vi "Transmit Messages with Rate-based Schedule.vi"() -> ()   [LabVIEW 2023]
doc: "This program opens the specified card, builds a transmit schedule \nusing transmit interval information in the channel configuration file,\nand then transmits the messages with changing data."
uses:
  <instrlib>/BTICardLib/Private/Initialize By Card Number and Core Number.vi
  <instrlib>/BTICardLib/Private/Configure Core From XML.vi
  <instrlib>/BTI429Lib/Private/Tx/Configure/Configure Tx Channel From XML.vi
  <instrlib>/BTI429Lib/Private/Core/Action-Status/Start Channel.vi
  <instrlib>/BTI429Lib/Private/Utility/Get BNR Sign.vi
  <instrlib>/BTI429Lib/Private/Utility/Get BNR Data.vi
  <instrlib>/BTI429Lib/Private/Utility/Get BNR Val.vi
  <instrlib>/BTI429Lib/Private/Utility/Get BNR Mantissa.vi
  <instrlib>/BTI429Lib/Private/Utility/Get BNR SSM.vi
  <instrlib>/BTI429Lib/Private/Utility/Set BNR Mantissa.vi
  <instrlib>/BTI429Lib/Private/Core/Action-Status/Stop Channel.vi
  <instrlib>/BTICardLib/BTICardLV.lvlib
  <instrlib>/BTI429Lib/BTI429LV.lvlib
panel:
  in  "Channel Configuration XML file name":string="Channel Config.xml"
  in  "Core Configuration XML file name":string="Core Config.xml"
  in  "Card Number":i32
  in  "Channel Number":i32=16
  in  "Core Number":i32
  out "Core Xml Path":path
  out "Channel Xml Path":path
  out "twosmantissaout":u32
  out "NEW sign out":u16
  in  "TwosComplement":u16
  out "message out":u32 format="%.0b"
  out "mantissa out":u32 format="%.0b"
  out "sign/status matrix (SSM)":u16 format="%1b"
  out "Data-NotSDI":u32 format="%.0b"
  out "MessageWithResosalution-NotSDI":string
  out "sign bit(29)":u16
  out "message-value":u32 format="%.0b"
  out "error out":errorcluster
  in  "stop":bool
  # "ARINC 429: Transmit Messages with Rate-based Schedule"
  # "©2016 Astronics Ballard Technology"
  # "This program opens the specified card, builds a transmit schedule \nusing transmit interval information in the channel configuration file,\nand the messages check."
  # "(parity(32)-ssm(31-30)-sign(29)-data(28-11)-sdi(10-9)-label(8-1))"
  # "(28-11bits)"
  # "IcludeSignBitBecause Arinc format is BNR(out(31-30))"
  # "Always Stop the card\nand Close the card when\ndone. Otherwise, the hardware\ncontinues to operate."
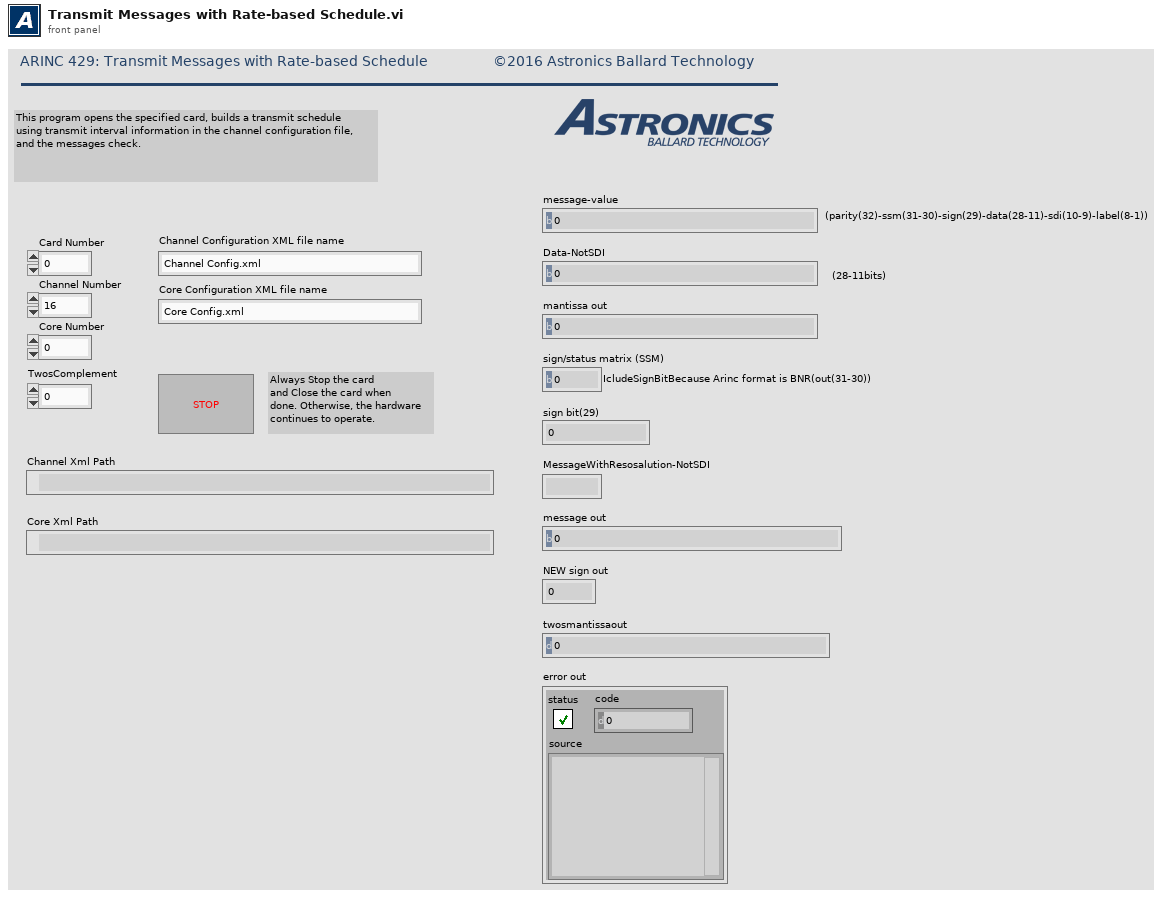
[diagram p1: front panel]
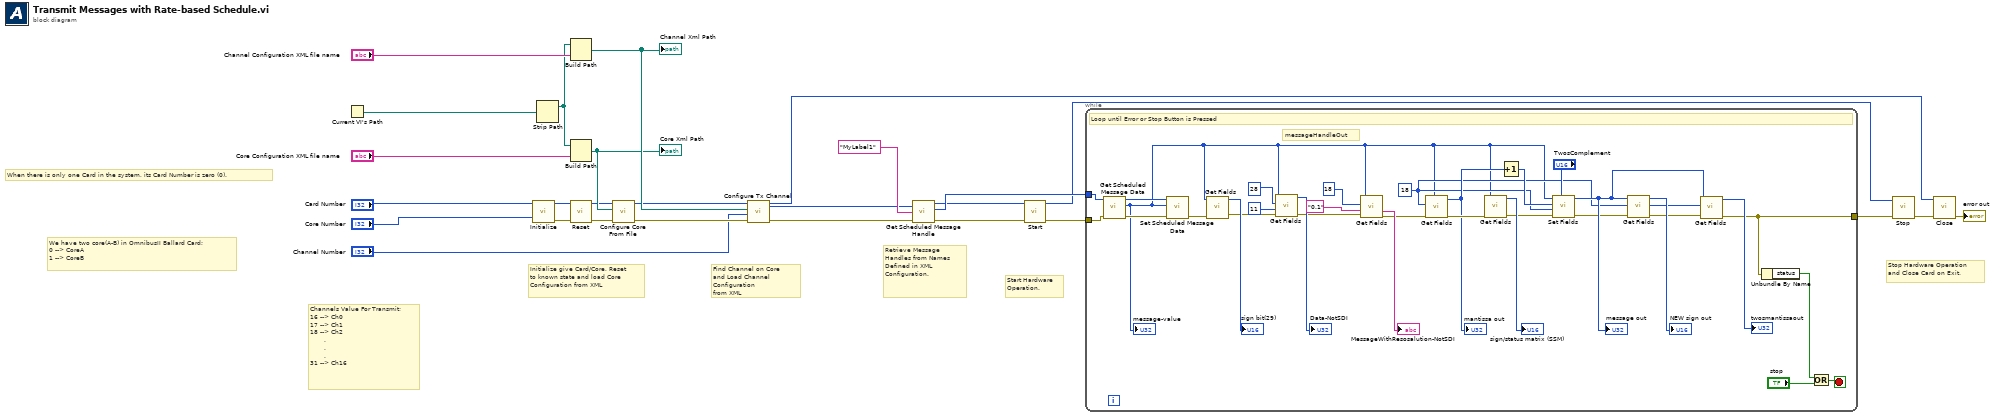
[diagram p0: block diagram]
diagram:
  # "We have two core(A-B) in OmnibusII Ballard Card;\n0 --> CoreA\n1 --> CoreB"
  # "When there is only one Card in the system, its Card Number is zero (0)."
  # "Channels Value For Transmit;\n16 --> Ch0\n17 --> Ch1\n18 --> Ch2\n       .\n       .\n       .\n31 --> Ch16"
  # "Stop Hardware Operation\nand Close Card on Exit."
  # "Start Hardware\nOperation."
  # "Retrieve Message Handles from Names\nDefined in XML Configuration."
  # "Find Channel on Core\nand Load Channel Configuration\nfrom XML"
  # "Initialize give Card/Core, Reset\nto known state and load Core\nConfiguration from XML"
  n1 = Current VI's Path() -> (path=w18:path)
  n2 = call-poly <instrlib>:"Initialize.vi"("core number"="Core Number", "card number"="Card Number") -> ("error out"=w12:errorcluster, "core handle out"=w13:u64)  [unwired: 8 in]
  n3 = Strip Path(path=w18) -> (stripped path=w8:path)  [unwired: 1 out]
  n4 = Build Path(base path=w8, name or relative path="Channel Configuration XML file name") -> (appended path=w17:path)
  "Channel Xml Path" <- w17
  n5 = Build Path(base path=w8, name or relative path="Core Configuration XML file name") -> (appended path=w14:path)
  "Core Xml Path" <- w14
  n6 = call <instrlib>:"Reset.vi"("error in (no error)"=w12, "core handle in"=w13) -> ("error out"=w10:errorcluster, "core handle out"=w11:u64)  [unwired: 8 in]
  n7 = call-poly <instrlib>:"Configure Core From File.vi"("error in (no error)"=w10, "configuration file path"=w14, "core handle in"=w11) -> ("error out"=w21:errorcluster, "core handle out"=w7:u64)  [unwired: 7 in]
  n8 = call-poly <instrlib>:"Configure Tx Channel.vi"("error in (no error)"=w21, "channel number in"="Channel Number", "configuration file path"=w17, "core handle in"=w7) -> ("error out"=w27:errorcluster, "channel handle out"=w22:u64, "core handle out"=w9:u64)  [unwired: 5 in]
  n9 = call <instrlib>:"Get Scheduled Message Handle.vi"("error in (no error)"=w27, "message name"="MyLabel1" ("msgname"), "channel handle in"=w22) -> ("error out"=w5:errorcluster, "message handle out"=w25:u64, "channel handle out"=w6:u64)  [unwired: 6 in]
  n10 = call-poly <instrlib>:"Start.vi"("error in (no error)"=w5, "channel handle in"=w6) -> ("error out"=w26:errorcluster, "channel handle out"=w20:u64)  [unwired: 8 in]
  n11 = while {
    tunnel: w26 -> [w33]
    tunnel: w25 -> [w34]
    tunnel: [w28] -> w4
    stop <- w37 stop-if-true
    w41 = u16 18 ("significant digits")
    # "messageHandleOut"
    # "Loop until Error or Stop Button is Pressed"
    n12 = call <instrlib>:"Get Scheduled Message Data.vi"("error in (no error)"=w33, "message handle in"=w34) -> ("error out"=w31:errorcluster, "value"=w29:u32, "message handle out"=w30:u64)  [unwired: 7 in]
    "message-value" <- w29
    n13 = call <instrlib>:"Set Scheduled Message Data.vi"("error in (no error)"=w31, "value"=w29, "message handle in"=w30) -> ("error out"=w32:errorcluster)  [unwired: 7 in, 1 out]
    n14 = call-poly <instrlib>:"Get Fields.vi"("error in (no error)"=w32, "message"=w29) -> ("error out"=w52:errorcluster, "sign out"=→"sign bit(29)":u16)  [unwired: 8 in]
    n15 = call-poly <instrlib>:"Get Fields.vi"("error in (no error)"=w52, "least significant bit"=u16 11, "most significant bit"=u16 28, "message"=w29) -> ("error out"=w51:errorcluster, "data out"=→"Data-NotSDI":u32)  [unwired: 6 in]
    n16 = call-poly <instrlib>:"Get Fields.vi"("error in (no error)"=w51, "resolution string"="0.1", "significant bits"=u16 18, "message"=w29) -> ("error out"=w49:errorcluster, "value out"=→"MessageWithResosalution-NotSDI":string)  [unwired: 6 in]
    n17 = call-poly <instrlib>:"Get Fields.vi"("error in (no error)"=w49, "significant digits"=w41, "message"=w29) -> ("error out"=w48:errorcluster, "mantissa out"=w45:u32)  [unwired: 7 in]
    "mantissa out" <- w45
    n18 = call-poly <instrlib>:"Get Fields.vi"("error in (no error)"=w48, "message"=w29) -> ("error out"=w47:errorcluster, "sign/status matrix (SSM) out"=→"sign/status matrix (SSM)":u16)  [unwired: 8 in]
    n19 = Increment(x=w45) -> (x+1=w44:u32)
    n20 = call-poly <instrlib>:"Set Fields.vi"("twos"="TwosComplement", "error in (no error)"=w47, "significant bits"=w41, "value"=w44, "message"=w29) -> ("error out"=w36:errorcluster, "message out"=w42:u32)  [unwired: 5 in]
    "message out" <- w42
    n21 = call-poly <instrlib>:"Get Fields.vi"("error in (no error)"=w36, "message"=w42) -> ("error out"=w35:errorcluster, "sign out"=→"NEW sign out":u16)  [unwired: 8 in]
    n22 = call-poly <instrlib>:"Get Fields.vi"("error in (no error)"=w35, "significant digits"=w41, "message"=w42) -> ("error out"=w28:errorcluster, "mantissa out"=→"twosmantissaout":u32)  [unwired: 7 in]
    n23 = Unbundle By Name(w28) -> ("status"=w39:bool)
    n24 = Or(x=w39, y="stop") -> (x .or. y?=w37:bool)
    n25 = Wait (ms)(milliseconds to wait=u32 200) -> ()  [unwired: 1 out]
  }
  n26 = call-poly <instrlib>:"Stop.vi"("error in (no error)"=w4, "channel handle in"=w20) -> ("error out"=w19:errorcluster)  [unwired: 8 in, 1 out]
  n27 = call <instrlib>:"Close.vi"("error in (no error)"=w19, "core handle in"=w9) -> ("error out"=→"error out":errorcluster)  [unwired: 8 in, 1 out]
